vi "Configure Notch Search.vi"(5 "State (T: Enable)":bool=TRUE, 7 "Notch Definition Value (-3.0)":dbl=-3.0, 8 "error in (no error)":errorcluster, 9 "Marker (1)":i32=1, 10 "Channel (1)":i32=1, 11 "VISA resource name":refnum<visa-resource-name>) -> (0 "error out":errorcluster, 3 "VISA resource name out":refnum<visa-resource-name>)   [LabVIEW 2018, in "Agilent ENA Series.lvlib"]
doc: "Configures the notch marker search.\n\nNotes:\n(1) This VI is not supported by E5070B, E5071B, and E5080A"
uses:
  Agilent ENA Series.lvlib
panel:
  # "Enable\n\nDisable"
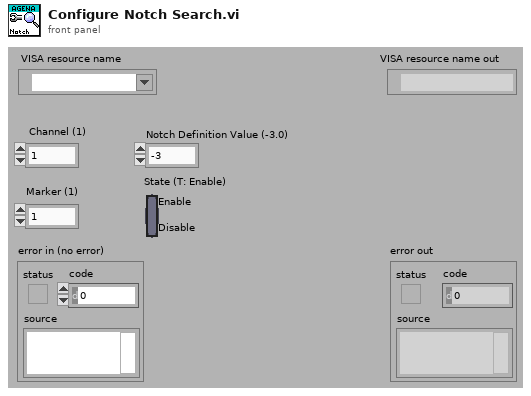
[diagram p1: front panel]
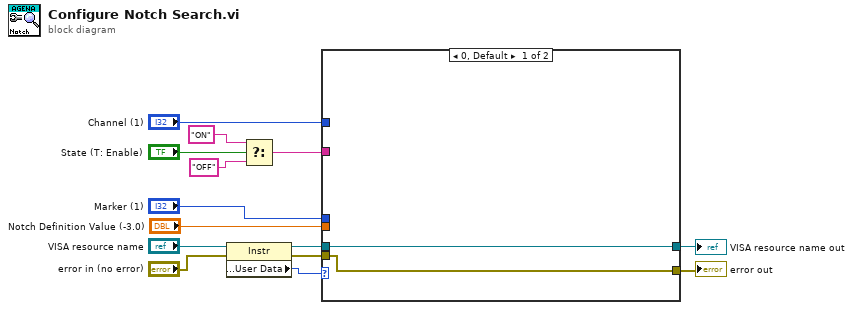
[diagram p0: block diagram]
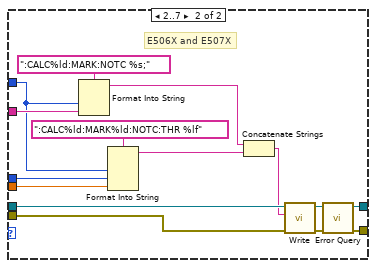
[diagram p2: hidden frame]
diagram:
  n1 = property class="Instr"(reference="VISA resource name", error in="error in (no error)") -> (reference out=w14:refnum<visa-resource-name>, error out=w13:errorcluster, "General Settings:User Data"=w12:u32)
  n2 = Select(t="ON", s="State (T: Enable)", f="OFF") -> (s? t:f=w5:string)
  n3 = case shown="0, Default" w12 {
    tunnel: w14 -> [w16 w31]
    tunnel: w13 -> [w15 w30]
    tunnel: [w16 w18] -> w2
    tunnel: [w15 w17] -> w1
    tunnel: "Channel (1)" -> [_ w26]
    tunnel: w5 -> [_ w28]
    tunnel: "Marker (1)" -> [_ w25]
    tunnel: "Notch Definition Value (-3.0)" -> [_ w24]
    frame 0, Default {
    }
    frame 2..7 {
      # "E506X and E507X"
      n4 = Format Into String(format string=":CALC%ld:MARK:NOTC %s;", w26, w28) -> (resulting string=w22:string)  [unwired: 2 in, 1 out]
      n5 = Format Into String(format string=":CALC%ld:MARK%ld:NOTC:THR %lf", w26, w25, w24) -> (resulting string=w23:string)  [unwired: 2 in, 1 out]
      n6 = Concatenate Strings(w22, w23) -> (w21:string)
      n7 = call "Write.vi"("error in (no error)"=w30, "String ()"=w21, "VISA resource name"=w31) -> ("error out"=w19:errorcluster, "VISA resource name out"=w20:refnum<visa-resource-name>)  [unwired: 6 in, 1 out]
      n8 = call "Error Query.vi"("error in (no error)"=w19, "VISA resource name"=w20) -> ("error out"=w17:errorcluster, "VISA resource name out"=w18:refnum<visa-resource-name>)  [unwired: 6 in, 2 out]
    }
  }
  "error out" <- w1
  "VISA resource name out" <- w2
